vi "triangle scan.vi"(11 "scan specification":T1) -> (2 "scan locations":u32[](array[numeric]), 3 "scan specification out":T1)   [LabVIEW 2010]
uses:
  scan_specification_tagResonant.ctl
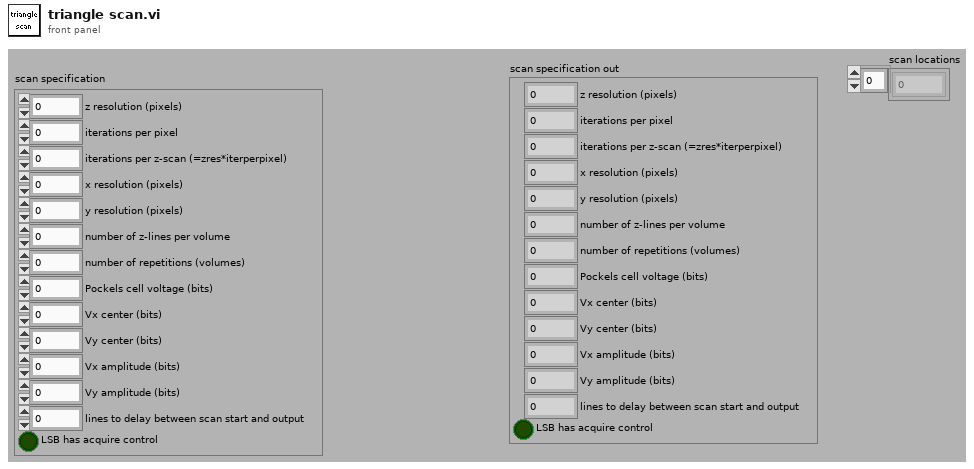
[diagram p1: front panel]
types:
  T1 = typedef "scan_specification_tagResonant.ctl" = cluster{"z resolution (pixels)":u16, "iterations per pixel":u16, "iterations per z-scan (=zres*iterperpixel)":u16, "x resolution (pixels)":u16, "y resolution (pixels)":u16, "number of z-lines per volume":u16, "number of repetitions (volumes)":i32, "Pockels cell voltage (bits)":i16, "Vx center (bits)":i16, "Vy center (bits)":i16, "Vx amplitude (bits)":i16, "Vy amplitude (bits)":i16, "lines to delay between scan start and output":u16, "LSB has acquire control":bool}
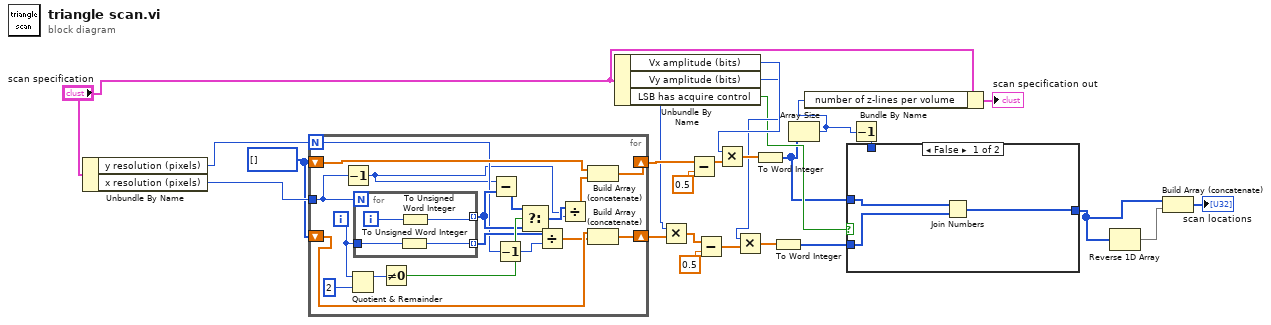
[diagram p0: block diagram]
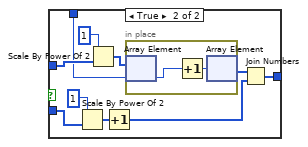
[diagram p2: hidden frame]
diagram:
  w22 = u16[] []
  n1 = Unbundle By Name("scan specification") -> ("y resolution (pixels)"=w23:u16, "x resolution (pixels)"=w24:u16)
  n2 = for {
    N: w23 -> [w27]
    tunnel: w24 -> [w30]
    shift-right: [w36] -> w21
    shift-left: w22 -> [w35]
    shift-right: [w34] -> w19
    shift-left: w22 -> [w33]
    i -> [w42]
    n3 = Decrement(x=w30) -> (x-1=w26:u16)
    n4 = Quotient & Remainder(x=w42, y=2) -> (x-y*floor(x/y)=w40:i32)  [unwired: 1 out]
    n5 = for {
      N: w30 -> [_]
      tunnel: [w44] -> w37 mode=indexing
      tunnel: w42 -> [w45]
      tunnel: [w43] -> w28 mode=indexing
      i -> [w46]
      n6 = To Unsigned Word Integer(number=w45) -> (unsigned 16bit integer=w43:u16)
      n7 = To Unsigned Word Integer(number=w46) -> (unsigned 16bit integer=w44:u16)
    }
    n8 = Not Equal To 0?(x=w40) -> (x != 0?=w39:bool)
    n9 = Subtract(x=w26, y=w37) -> (x-y=w38:u16[])
    n10 = Decrement(x=w27) -> (x-1=w25:i32)
    n11 = Select(t=w38, s=w39, f=w37) -> (s? t:f=w31:u16[])
    n12 = Divide(x=w28, y=w25) -> (x/y=w29:dbl[])
    n13 = Divide(x=w31, y=w26) -> (x/y=w32:dbl[])
    n14 = Build Array (concatenate)(w35, w32) -> (w36:dbl[])
    n15 = Build Array (concatenate)(w33, w29) -> (w34:dbl[])
  }
  n16 = Unbundle By Name("scan specification") -> ("Vx amplitude (bits)"=w20:i16, "Vy amplitude (bits)"=w10:i16, "LSB has acquire control"=w9:bool)
  n17 = Multiply(x=w10, y=w19) -> (x*y=w14:dbl[])
  n18 = Subtract(x=w21, y=0.5) -> (x-y=w17:dbl[])
  n19 = Subtract(x=w14, y=0.5) -> (x-y=w11:dbl[])
  n20 = Multiply(x=w20, y=w17) -> (x*y=w13:dbl[])
  n21 = Multiply(x=w10, y=w11) -> (x*y=w12:dbl[])
  n22 = To Word Integer(number=w13) -> (16bit integer=w8:i16[])
  n23 = To Word Integer(number=w12) -> (16bit integer=w7:i16[])
  n24 = Array Size(array=w8) -> (size(s)=w6:i32)
  n25 = Bundle By Name(cluster="scan specification", "number of z-lines per volume"=w6) -> (→"scan specification out":T1)
  n26 = Decrement(x=w6) -> (x-1=w5:i32)
  n27 = case shown="False" w9 {
    tunnel: w8 -> [w49 w55]
    tunnel: w7 -> [w48 w59]
    tunnel: w5 -> [_ w53]
    tunnel: [w47 w50] -> w3
    frame False {
      n28 = Join Numbers(hi=w49, lo=w48) -> ((hi.lo)=w47:u32[])
    }
    frame True {
      n29 = Scale By Power Of 2(n=1, x=w59) -> (x*2^n=w57:i16[])
      n30 = Scale By Power Of 2(n=1, x=w55) -> (x*2^n=w54:i16[])
      n31 = Increment(x=w57) -> (x+1=w51:i16[])
      n32 = in-place {
        n33 = in-place-array #1(w54, w53) -> (w61:i16)
        n34 = Increment(x=w61) -> (x+1=w60:i16)
        n35 = in-place-array #1(w60) -> (w52:i16[])  [unwired: 1 out]
      }
      n36 = Join Numbers(hi=w52, lo=w51) -> ((hi.lo)=w50:u32[])
    }
  }
  n37 = Reverse 1D Array(array=w3) -> (reversed array=w4:u32[])
  n38 = Build Array (concatenate)(w3, w4) -> (→"scan locations":u32[])
